vi "4 DDS.vi"(8 "input valid":bool=TRUE, 9 "pdw in":T2 {"frequency shift" format="%#_12f"}, 10 "free DDS before me?":bool, 11 "new PDW in":bool) -> (0 "output valid":bool, 1 "state of every DDS":bool[](array[boolean]), 2 "have free DDS":bool, 3 "IQ out":T1)   [LabVIEW 2021]
doc: "transmit pulse with one free DDS inside.\nmust have no DDS before him (the distribute is to give the lowest mun DDS the pulse)"
uses:
  pulse_tx_vis/pdw.ctl
  pulse_tx_vis/mode_type.ctl
  <instrlib>/_niInstr/DSP/v1/Shared/Public/IQ Data.ctl
  <instrlib>/_niInstr/DSP/v1/Shared/niInstr DSP v1 Shared.lvlib
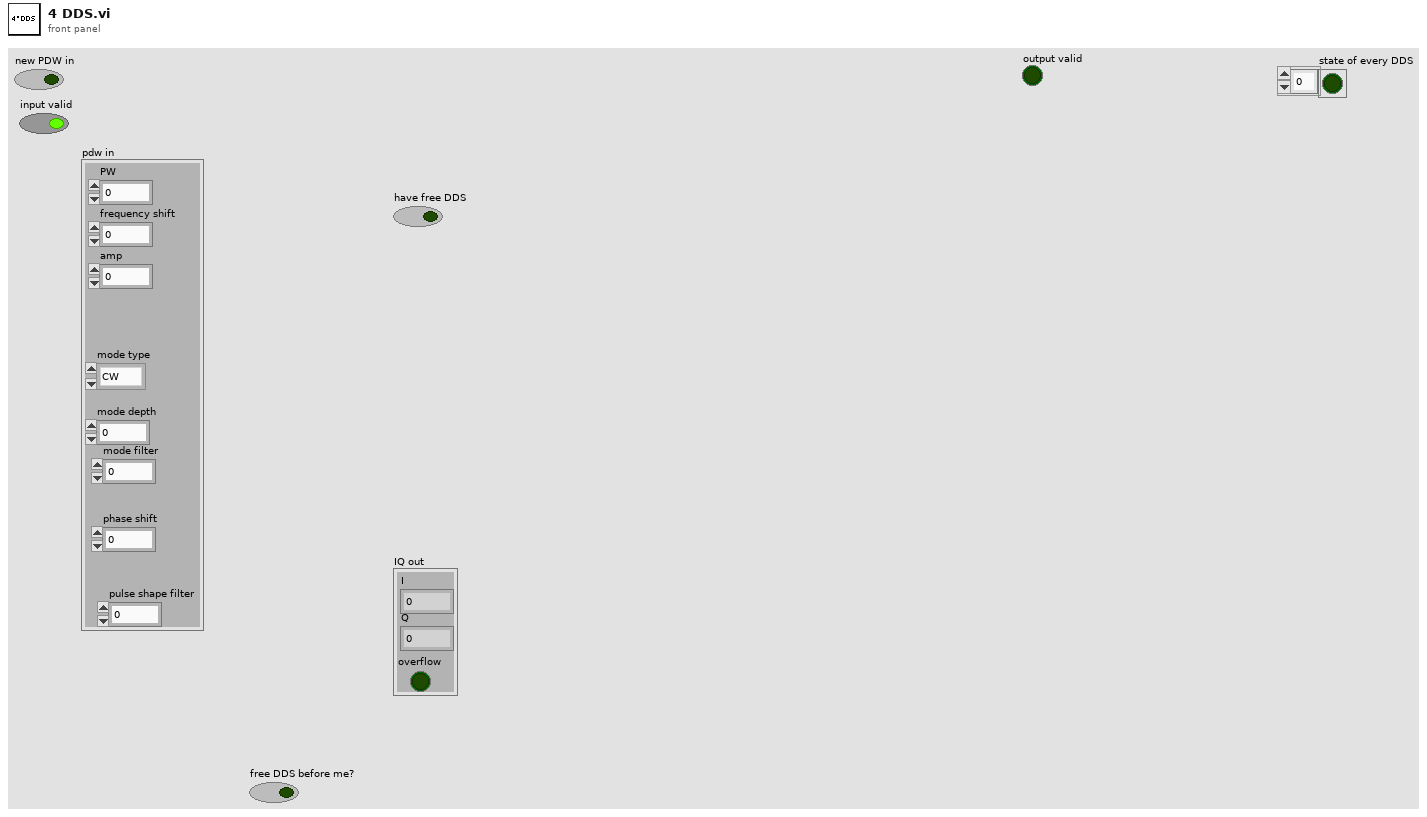
[diagram p1: front panel]
types:
  T1 = typedef "niInstr DSP v1 Shared.lvlib/IQ Data.ctl" = cluster{"I":fxp<+/-,18,1>, "Q":fxp<+/-,18,1>, "overflow":bool}
  T2 = typedef "pdw.ctl" = cluster{"PW":u32, "frequency shift":fxp<+/-,48,0>, "amp":fxp<+/-,18,1>, "mode type":T3, "mode depth":u32, "mode filter":u8, "phase shift":fxp<+/-,16,1>, "pulse shape filter":u8}
  T3 = typedef "mode_type.ctl" = enum8{"CW", "NC - CW", "NC - cw", "LFM", "BPSK", "QPSK"}
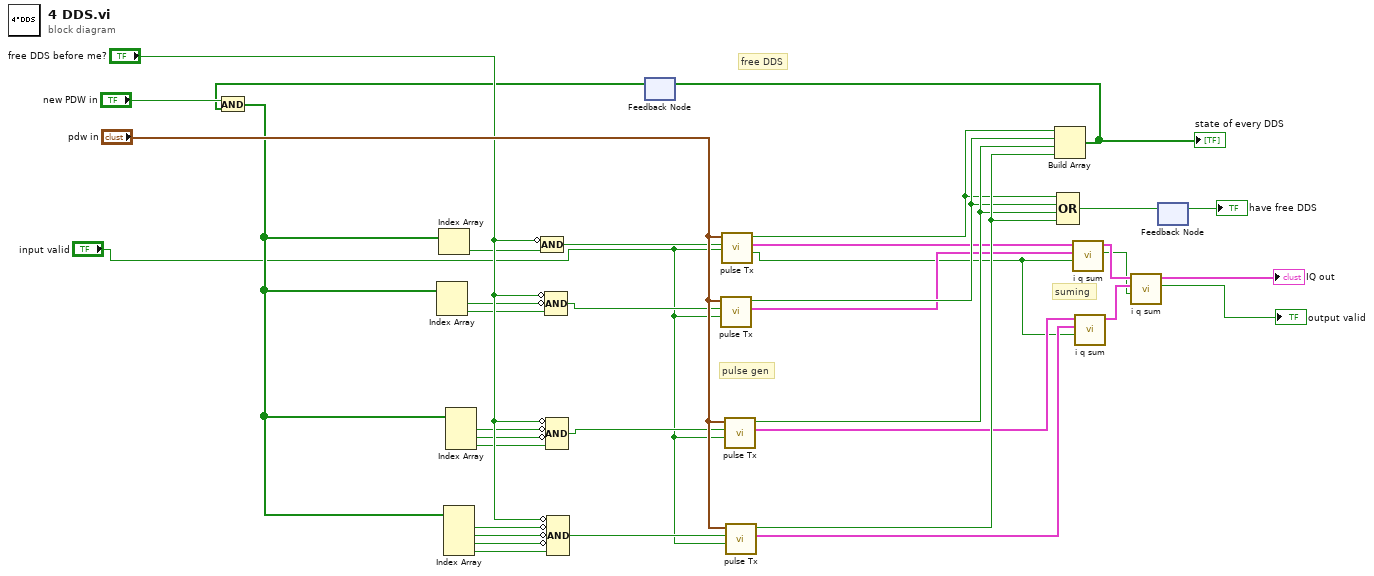
[diagram p0: block diagram]
diagram:
  # "free DDS"
  # "suming"
  # "pulse gen"
  n1 = feedback #1() -> (w8:bool[])  [unwired: 1 in]
  n2 = And(x="new PDW in", y=w8) -> (x .and. y?=w7:bool[])
  n3 = Index Array(array=w7) -> (element #1=w21:bool, element #2=w19:bool)  [unwired: 2 in]
  n4 = Index Array(array=w7) -> (element=w17:bool)  [unwired: 1 in]
  n5 = Index Array(array=w7) -> (element #1=w29:bool, element #2=w28:bool, element #3=w27:bool, element #4=w26:bool)  [unwired: 4 in]
  n6 = Index Array(array=w7) -> (element #1=w25:bool, element #2=w24:bool, element #3=w23:bool)  [unwired: 3 in]
  n7 = Compound Arithmetic op=AND(invert "free DDS before me?", w17) -> (w18:bool)
  n8 = Compound Arithmetic op=AND(invert "free DDS before me?", invert w21, w19) -> (w20:bool)
  n9 = Compound Arithmetic op=AND(invert "free DDS before me?", invert w25, invert w24, w23) -> (w22:bool)
  n10 = Compound Arithmetic op=AND(invert "free DDS before me?", invert w29, invert w28, invert w27, w26) -> (w30:bool)
  n11 = call "pulse Tx.vi"("enable line"="input valid", "take it!"=w20, "Cluster"="pdw in") -> ("data out"=w14:T1, "free dds"=w33:bool)  [unwired: 4 in, 3 out]
  n12 = call "pulse Tx.vi"("enable line"="input valid", "take it!"=w18, "Cluster"="pdw in") -> ("output valid"=w3:bool, "data out"=w13:T1, "free dds"=w32:bool)  [unwired: 4 in, 2 out]
  n13 = call "pulse Tx.vi"("enable line"="input valid", "take it!"=w22, "Cluster"="pdw in") -> ("data out"=w15:T1, "free dds"=w34:bool)  [unwired: 4 in, 3 out]
  n14 = call "pulse Tx.vi"("enable line"="input valid", "take it!"=w30, "Cluster"="pdw in") -> ("data out"=w16:T1, "free dds"=w35:bool)  [unwired: 4 in, 3 out]
  n15 = Build Array(w32, w33, w34, w35) -> (w10:bool[])
  "state of every DDS" <- w10
  n16 = feedback-in #1(w10) -> ()
  n17 = Compound Arithmetic op=OR(w32, w33, w34, w35) -> (w6:bool)
  n18 = call "i q sum.vi"("input valid"=w3, 10:"data in"=w14, 11:"data in"=w13) -> ("output valid"=w2:bool, "output cluster"=w12:T1)  [unwired: 7 in]
  n19 = call "i q sum.vi"("input valid"=w3, 10:"data in"=w16, 11:"data in"=w15) -> ("output cluster"=w11:T1)  [unwired: 7 in, 1 out]
  n20 = call "i q sum.vi"("input valid"=w2, 10:"data in"=w11, 11:"data in"=w12) -> ("output valid"=→"output valid":bool, "output cluster"=→"IQ out":T1)  [unwired: 7 in]
  n21 = feedback #2() -> (→"have free DDS":bool)  [unwired: 1 in]
  n22 = feedback-in #2(w6) -> ()
